vi "grabber_v2.vi"() -> ()   [LabVIEW 2010]
uses:
  <vilib>/Platform/TimedLoop/XDataNode/XDataNode.xnode
  <vilib>/Platform/TimedLoop/XDataNode/wakeup.ctl
  <vilib>/Platform/TimedLoop/XDataNode/XDNodeRunTimeDep.lvlib
  <vilib>/Platform/TimedLoop/XDataNode/nitl_modes.ctl
  <vilib>/Platform/TimedLoop/XDataNode/timing_clust.ctl
  <vilib>/rvi/interface/nirviCloseFPGA/nirviCloseFPGA.xnode
  <vilib>/rvi/interface/nirviMethod/nirviMethod.xnode
  <vilib>/rvi/interface/nirviReadWriteControl/nirviReadWriteControl.xnode
  <vilib>/Utility/error.llb/Error Cluster From Error Code.vi
  <vilib>/rvi/errors/niLvFpgaWhatHappensToTopLevelVI.ctl
  <vilib>/rvi/interface/common/niFpgaNodeNameForErrorReporting.ctl
  <vilib>/rvi/errors/niLvFpgaAdjustHostInterfaceError.vi
  <vilib>/dex/Flush And Wait Empty Condition.ctl
  NiFpgaLv.dll
  C:/Program Files (x86)/National Instruments/LabVIEW 2010/Targets/NI/FPGA/StockFPGA_IntfPrivate/ScriptTemplates/StockFPGA_ReadBigControlPlusUnflatten.vi
  <vilib>/FPGAPlugInAG/Dynamic/niLvFpga_Read32_Dynamic.vi
  C:/Program Files (x86)/National Instruments/LabVIEW 2010/Targets/NI/FPGA/StockFPGA_IntfPrivate/ScriptTemplates/StockFPGA_InlinedAdjustErrorForReadWrite.vi
  <vilib>/FPGAPlugInAG/Dynamic/niLvFpga_Close_Dynamic.vi
  config_data_cluster.ctl
panel:
  out "data lost":bool
  out "scan sum":T1
  out "y galvo feedback":i16(graph)
  out "x galvo feedback":i16(graph)
  out "z value":i16
  out "y value":i16
  out "x value":i16
  out "center of mass":cluster{"x avg":i16, "y avg":i16, "z avg":i16}
  in  "turn on displays":bool
  in  "Mark fly-forward phase?":bool
  in  "adjust N sums":u32=100 max=10000 step=20
  in  "fake image fast loop?":bool
  in  "Transpose graph view?":bool
  in  "Display green and red PMT?":bool
  in  "pick last TAG slice":u32
  in  "pick first TAG slice":u32
  in  "choose TAG slice?":bool
  out "ch1:position X":dbl
  out "ch0:position X":dbl
  in  "Adjust TAG phase":bool
  out "TAG profile at position X":dbl[][](graph)
  out "channel1":dbl[][](graph)
  out "channel0":dbl[][](graph)
  in  "N sums":u32(slide)=10 scale=0.0..100.0
  out "loop time":u32
  out "x galvo":i16(graph)
  out "scan specification":T2={"x amplitude"=100, "x resolution (pixels)"=28, "x offset fly-forward (iterations)"=50, "x offset fly-back (iterations)"=100, "y resolution (nr. of lines)"=80, "y step size"=30, "iterations per pixel"=5, "number of frames"=-1, "y offset (pixels)"=0, "number of y-brake lines  (before y-fly-back)"=0, "number y-brake lines (after y-fly-back)"=40, "number of y-fly-back steps"=0, "lines per z step"=1, "number of z/intensity tuples"=228, "number of repetitions (volumes or planes)"=-1, "z step size derived"=32, "choose the beginning of z scan"=FALSE, "number of frames (settings)"=80, "FPGA trajectory?"=TRUE, "Pockels cell voltage (bits)"=0, "Vy min(bits)"=0, "Vz min(bits)"=0}
  out "channel data block 2":dbl[][](graph)
  in  "fake image?":bool
  in  "xy view?":bool
  in  "Pockels cell voltage":i16(slide) min=-750 max=750 step=5 scale=-750.0..750.0
  out "DAC voltages":T3
  out "no. of extra wait lines written to FPGA FIFO":i32
  out "no. of z/int tuples written to FPGA FIFO":i32
  out "number of update commands received":i32
  out "extra wait lines set":bool
  out "zIntensity tuples set":bool
  out "scan spec set":bool
  out "display loop finished":bool
  in  "stop acquisition at FIFO overflow?  GRABBER":bool
  out "acquire?":bool
  out "FIFO overflow":bool
  out "scan":bool
  out "stop FPGA":bool
  out "wait for trigger?":bool
  out "stop acquisition at FIFO overflow?":bool
  out "scanning? FPGA":bool
  out "counter cluster out":T4
  out "extra waitlines array entries":u32[](graph)
  out "extra waitlines received by FPGA":u32
  out "no. of extra waitlines received":i32
  out "no of correctly transferred z tuples":u32
  out "z-points transfer corrupt?":bool
  out "intensity values":u16[](graph)
  out "z values":u16[](graph)
  out "no. of z/int. tubles received":i32
  out "z/intensity tuples received by FPGA":u32
  in  "wait till update":u32=500
  out "configuration":T5
  out "read FIFO overflow duration [ms]":u32
  out "read pixels duration [ms]":u32
  out "stream pixels [ms]":u32
  in  "Close front-panel?":bool=TRUE
  out "initialised?":bool
  in  "stop":bool
  out "command lp err":errorcluster
  out "error out":errorcluster
  out "effective read-block size":u32
  in  "max read block size":u32=32000
  out "read loop ctr":i32
  out "pixels read from FPGA":u64
  out "elements in FPGA FIFO":u32
  out "last received command":string
  out "command loop finished":bool
  out "read loop finished":bool
  out "scanning?":bool
  out "FIFO overflow?":bool
  out "data read from FPGA FIFO":u32[](array[numeric])
  # "enter a number between -+750V"
  # "Sum a single frame N times before displaying:"
  # "ms"
  # "automatically sets N=100 sums, otherwise FPGA buffer overflow"
  # "When T: displays and saves ch0.bin= green and ch1.bin =red\nWhen F: displays and saves ch0.bin= greenFF  and ch1.bin= greenFB  (FF=fly-forward and FB=fly-back)"
  # "Use when you want to display and save green and red PMT with marked FF and FB phases\nWhen T: fly-forward=photon counts+2^15 (number 1 at U16's most significant value)\n               and fly-back=photon counts\nWhen F: saves true photon count in both FF and FB phases of the red and green channel"
  # "How to use:\nTo adjust TAG phase\n1. set \"xy gavlo view?\"=F\n2. adjust Tag phase? = T\n3. drag cursor to desired x position\n   -- indicator below\n4. check z profile on the graph\n5. when done set N=0"
  # "How to use:\n1. set \"xy gavlo view?\"=T\n    on the main HS window\n2. to display xy view, sum all z stacks\n          set xy view?=T\n3. to choose a range of z slices to sum\na) xy view?=T\nb)choose TAG slice?=T\nc)eg. pick first Tag slice=3, pick last TAG slice=5\n   -> sums 3+4+5\nd) to display just one slice \n     set \"first=last\""
  # "RealTime Grabber"
  # "Status"
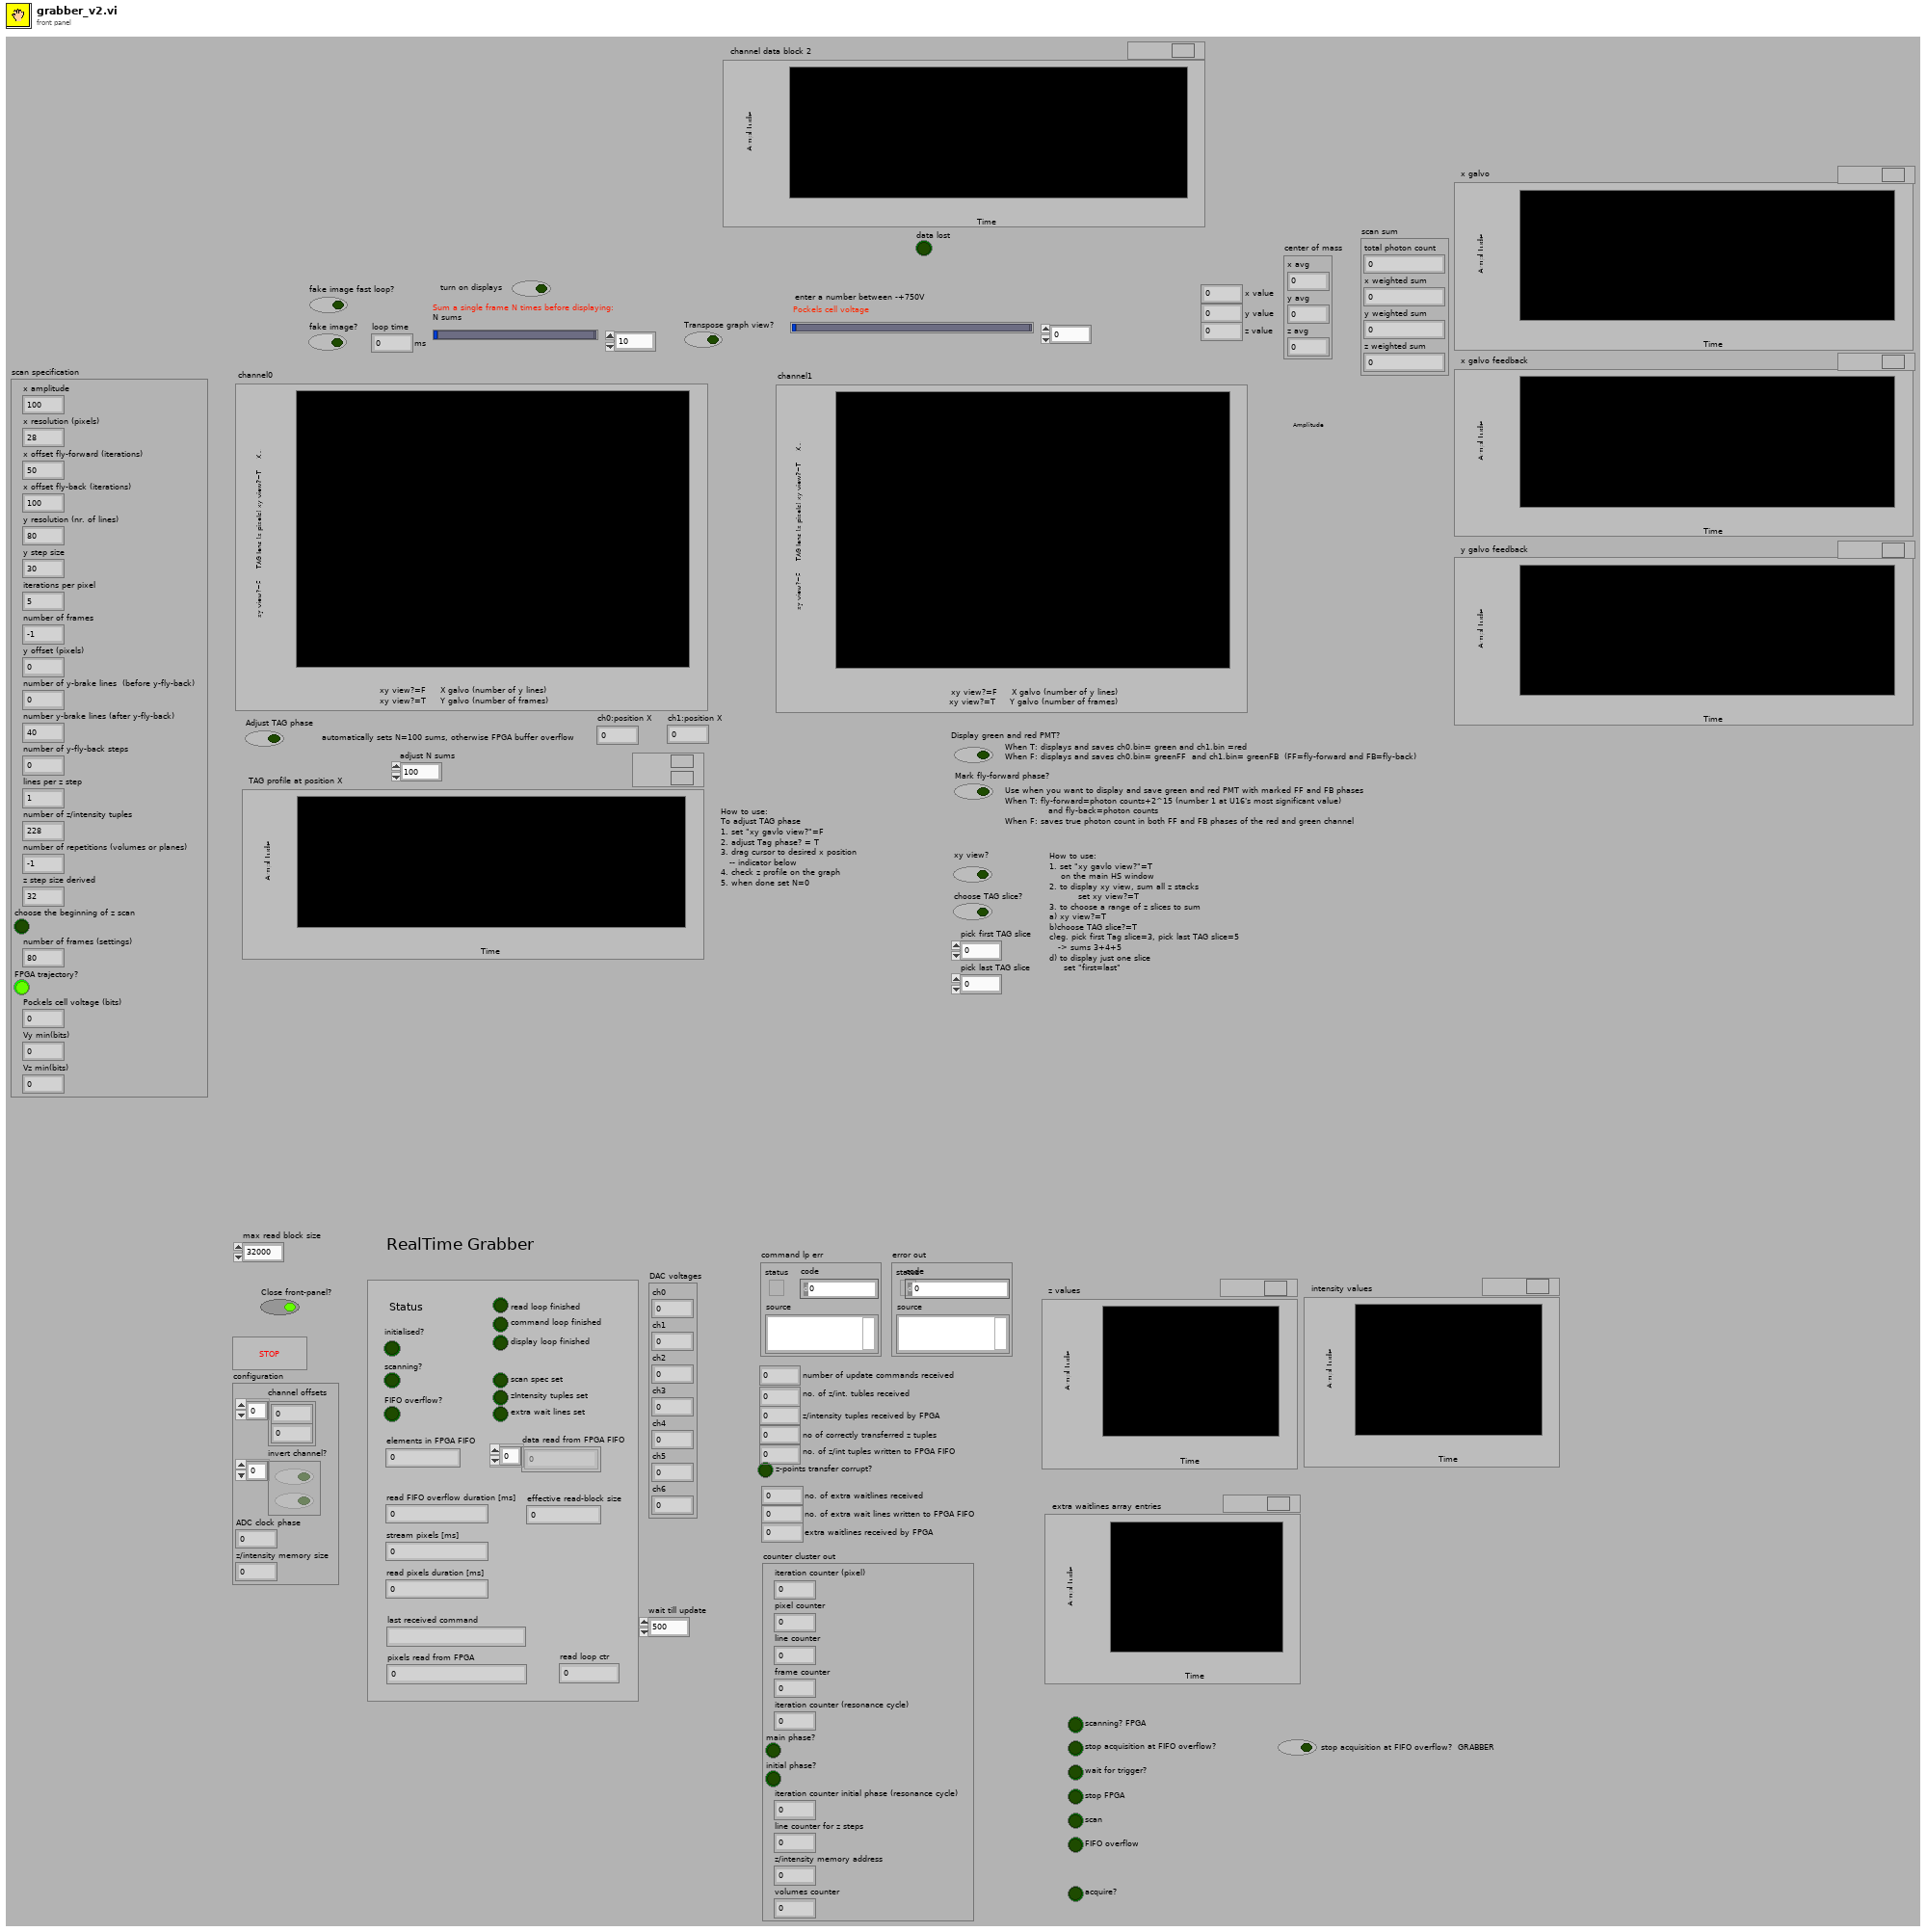
[diagram p1: front panel]
types:
  T1 = cluster{"total photon count":u64, "x weighted sum":i64, "y weighted sum":i64, "z weighted sum":i64}
  T2 = cluster{"x amplitude":u16, "x resolution (pixels)":u16, "x offset fly-forward (iterations)":u16, "x offset fly-back (iterations)":u16, "y resolution (nr. of lines)":u16, "y step size":u16, "iterations per pixel":u16, "number of frames":i32, "y offset (pixels)":u16, "number of y-brake lines  (before y-fly-back)":u16, "number y-brake lines (after y-fly-back)":u16, "number of y-fly-back steps":u16, "lines per z step":u16, "number of z/intensity tuples":u16, "number of repetitions (volumes or planes)":i32, "z step size derived":u16, "choose the beginning of z scan":bool, "number of frames (settings)":i32, "FPGA trajectory?":bool, "Pockels cell voltage (bits)":i16, "Vy min(bits)":i16, "Vz min(bits)":i16}
  T3 = cluster{"ch0":u16, "ch1":i16, "ch2":i16, "ch3":i16, "ch4":u16, "ch5":u16, "ch6":u16}
  T4 = cluster{"iteration counter (pixel)":u16, "pixel counter":u16, "line counter":u16, "frame counter":u16, "iteration counter (resonance cycle)":u16, "main phase?":bool, "initial phase?":bool, "iteration counter initial phase (resonance cycle)":u16, "line counter for z steps":u16, "z/intensity memory address":u32, "volumes counter":u16}
  T5 = typedef "config_data_cluster.ctl" = cluster{"channel offsets":u32[], "invert channel?":bool[], "ADC clock phase":i32, "z/intensity memory size":i32}
  T6 = cluster{"volumeQueue":refnum<queue>, "lineQueue":refnum<queue>, "comQueue":refnum<queue>}
  T7 = typedef "network_streaming_queues_cluster.ctl" = cluster{"data writer endpoint":refnum<k21>, "command reader endpoint":refnum<k21>, "settings reader endpoint":refnum<k21>, "z/intensity tuples reader endpoint":refnum<k21>, "extra waitlines reader endpoint":refnum<k21>}
  T8 = typedef "XDNodeRunTimeDep.lvlib/timing_clust.ctl" = cluster{"Expected End [f-1]":u64, "Actual End [f-1]":u64, "Finished Late? [f-1]":bool, "Expected End [i-1]":u64, "Actual End [i-1]":u64, "Finished Late? [i-1]":bool, "Expected Start [i]":u64, "Actual Start [i]":u64, "Expected Start [f]":u64, "Actual Start [f]":u64, "Source Name":string, "Structure Name":string, "Period":i64, "Deadline":i64, "Offset":i64, "Start":i64, "Priority":i32, "Timeout":i32, "Mode":T9, "Wakeup Reason":T10, "Error":errorcluster, "Source Type":string, "Secondary Source Type":string, "Global End Time":u64, "Global Start Time":u64, "Frame Duration":u64, "Iteration Duration":u64, "Assigned CPU":i32, "I/O Scan Engine Mode":u32}
  T9 = typedef "XDNodeRunTimeDep.lvlib/nitl_modes.ctl" = enum32{"No Change", "Process missed periods, maintain original phase", "Discard missed periods, maintain original phase", "Process missed periods, ignore original phase", "Discard missed periods, ignore original phase"}
  T10 = typedef "XDNodeRunTimeDep.lvlib/wakeup.ctl" = enum32{"Normal", "Aborted", "Asynchronous wakeup", "Timing source error", "Timed loop error", "Timeout"}
  T11 = typedef "niFpgaNodeNameForErrorReporting.ctl" = enum16{"Open FPGA VI Reference", "Read/Write Control", "Invoke Method: Abort", "Invoke Method: Acknowledge IRQ", "Invoke Method: Download", "Invoke Method: FIFO.Configure", "Invoke Method: FIFO.Read", "Invoke Method: FIFO.Start", "Invoke Method: FIFO.Stop", "Invoke Method: FIFO.Write", "Invoke Method: Reset", "Invoke Method: Run", "Invoke Method: Wait on IRQ", "Close FPGA VI Reference"}
  T12 = typedef "niLvFpgaWhatHappensToTopLevelVI.ctl" = enum16{"top level VI scripted behind XNode", "top level VI inlined behind XNode"}
  T13 = typedef "Flush And Wait Empty Condition.ctl" = u8
  T14 = typedef "scan_specification_cluster.ctl" = cluster{"x amplitude":u16, "x resolution (pixels)":u16, "x offset fly-forward (iterations)":u16, "x offset fly-back (iterations)":u16, "y resolution (nr. of lines)":u16, "y step size":u16, "iterations per pixel":u16, "number of frames":i32, "y offset (pixels)":u16, "number of y-brake lines  (before y-fly-back)":u16, "number y-brake lines (after y-fly-back)":u16, "number of y-fly-back steps":u16, "lines per z step":u16, "number of z/intensity tuples":u16, "number of repetitions (volumes or planes)":i32, "z step size derived":u16, "choose the beginning of z scan":bool, "number of frames (settings)":i32, "FPGA trajectory?":bool, "Pockels cell voltage (bits)":i16, "Vy min(bits)":i16, "Vz min(bits)":i16}
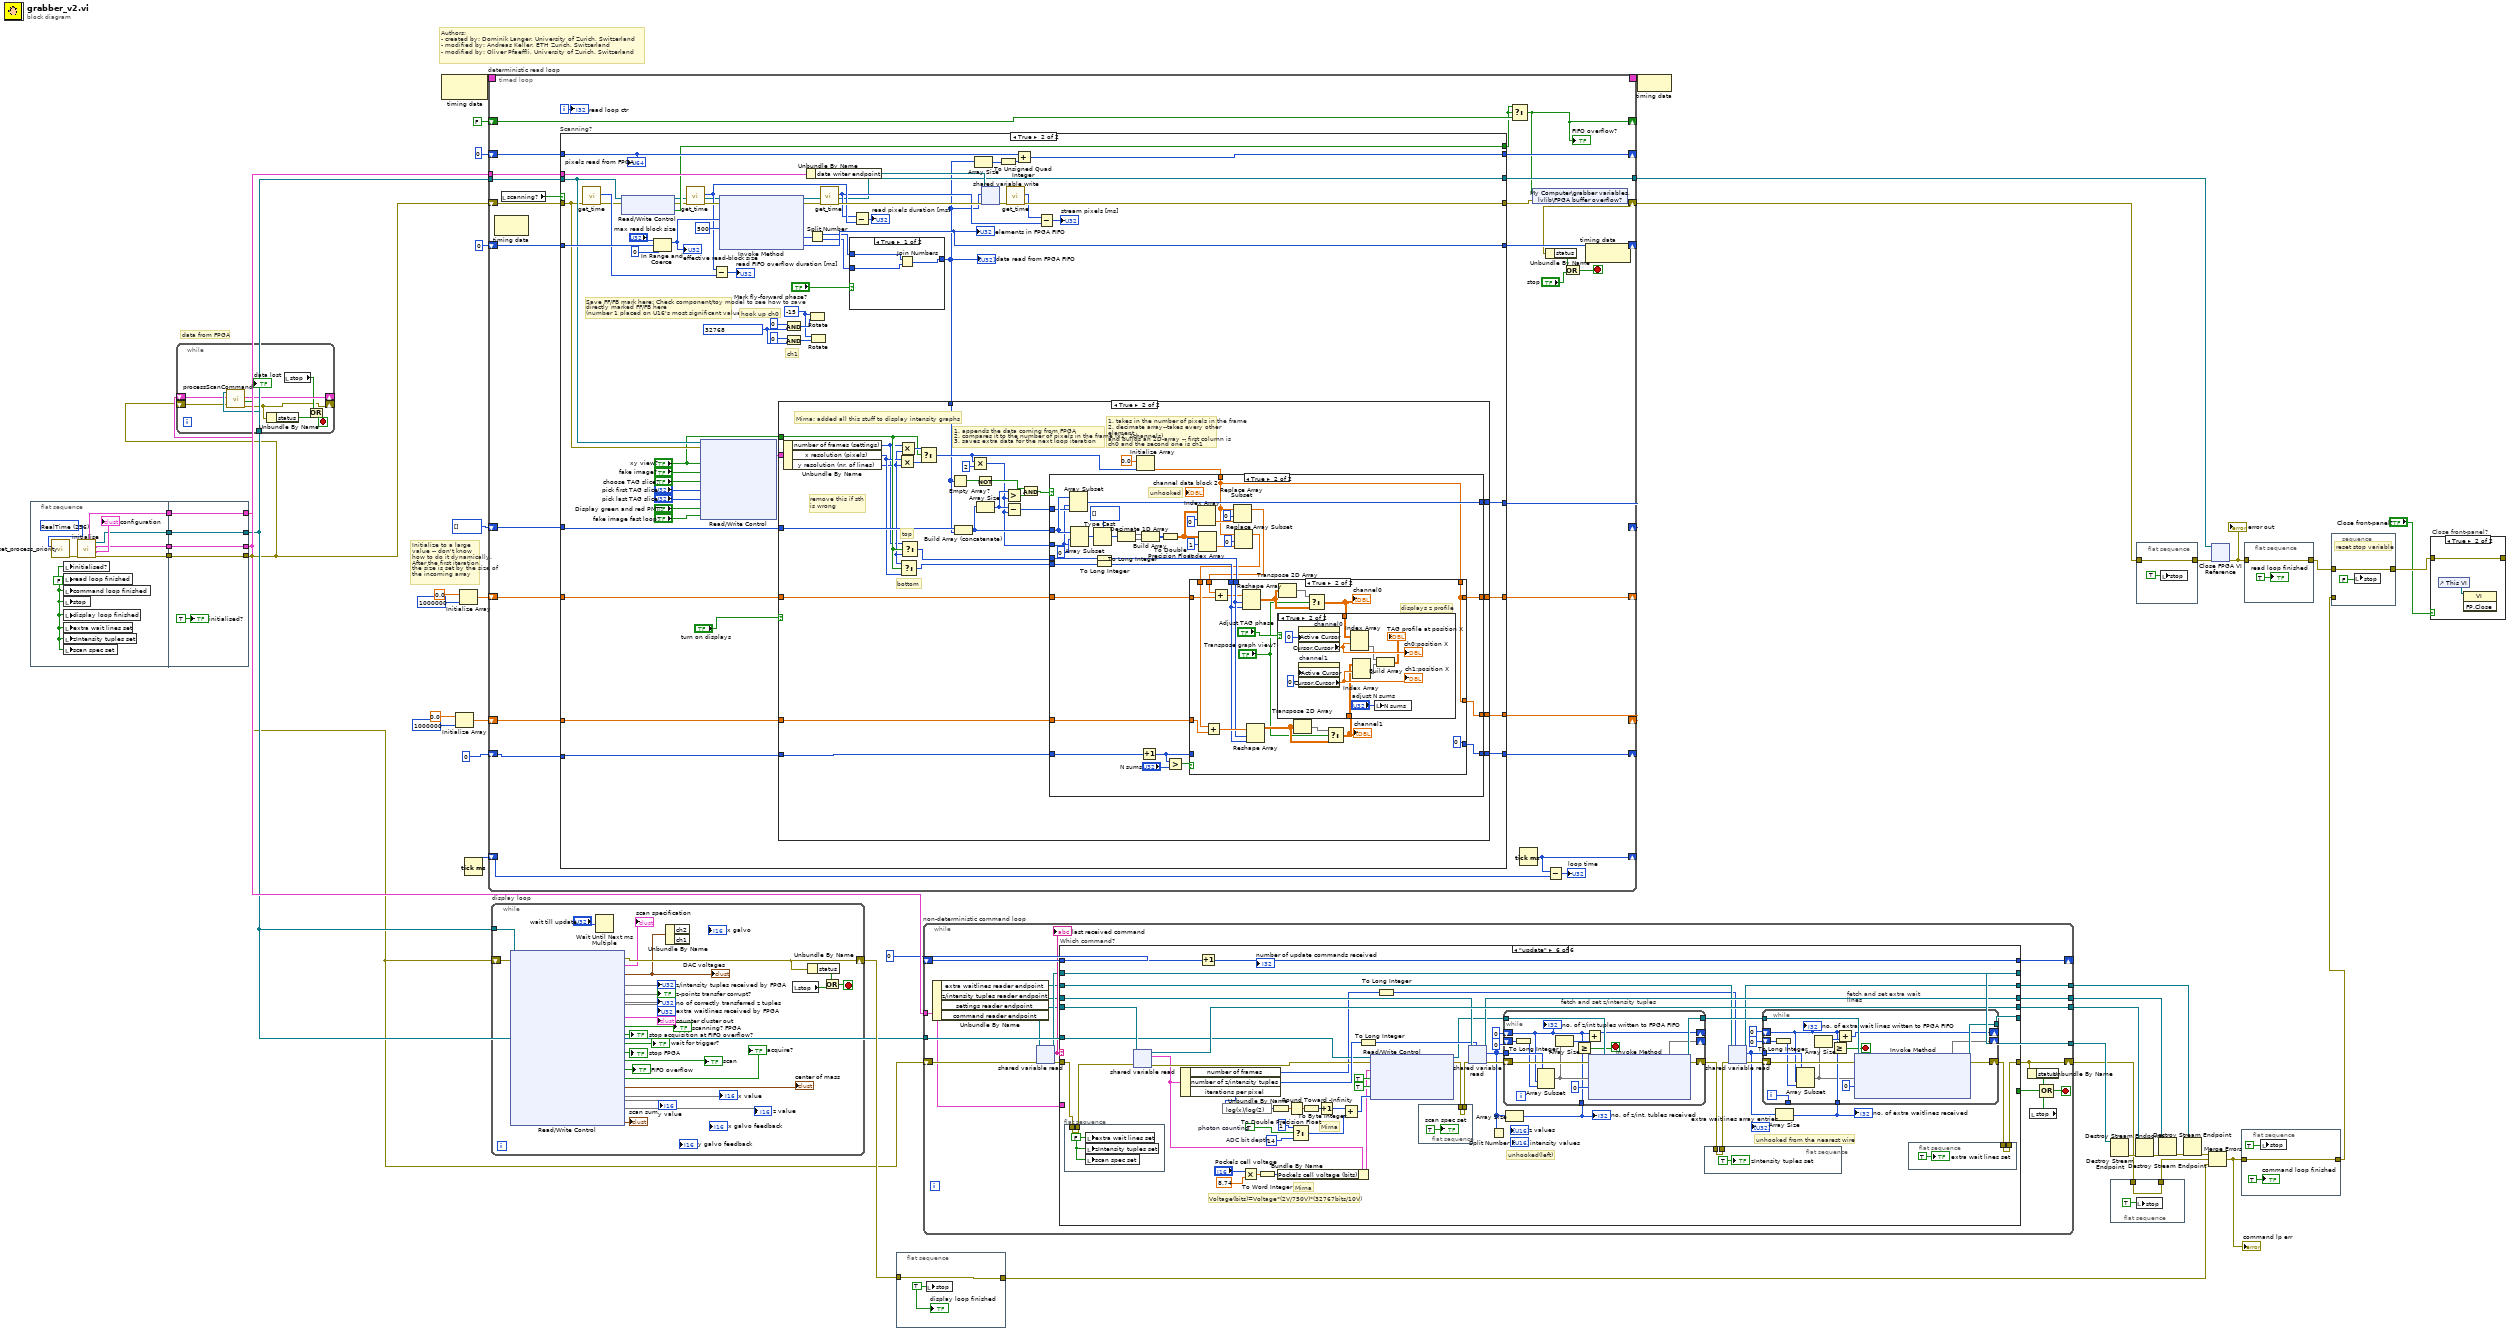
[diagram p0: block diagram]
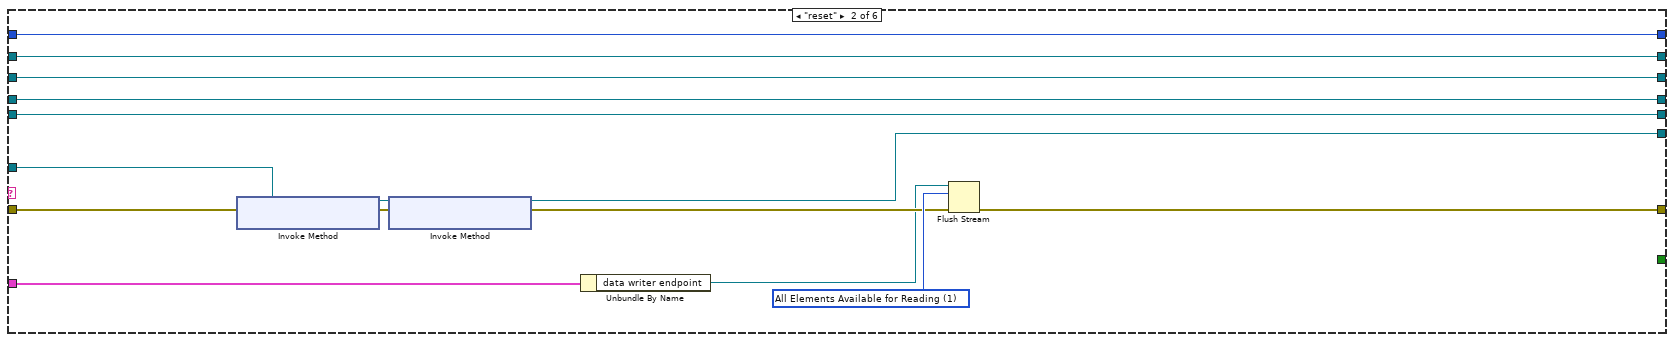
[diagram p4: hidden frame]
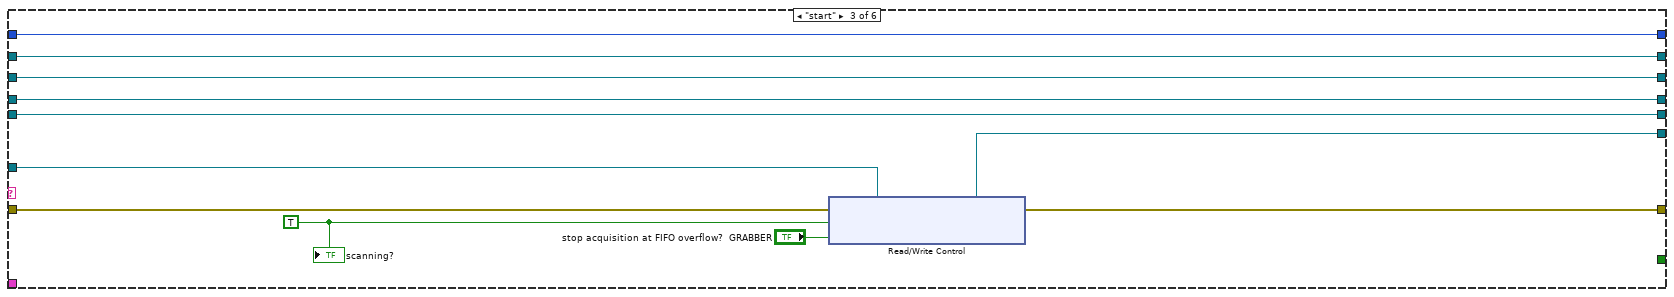
[diagram p5: hidden frame]
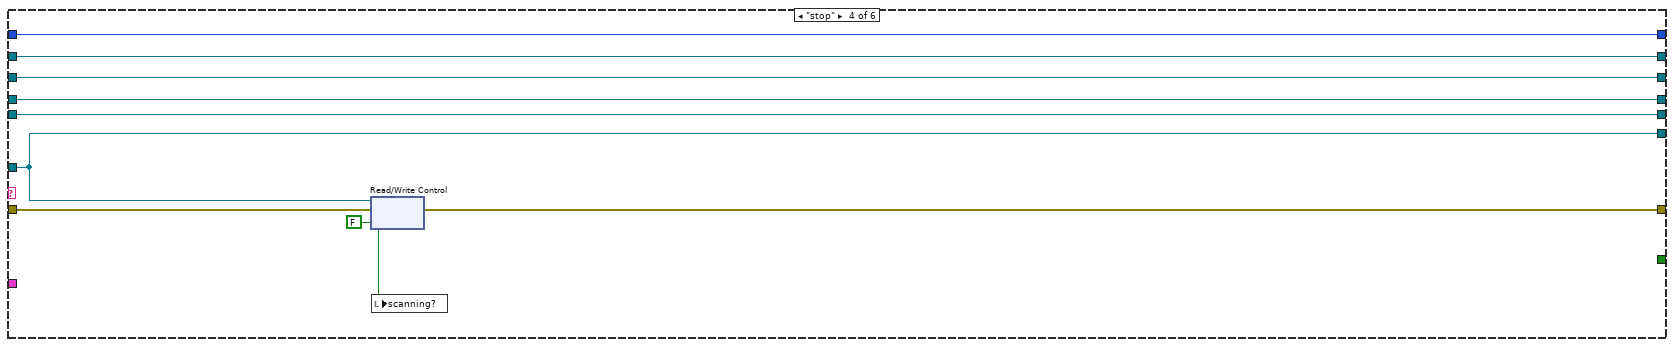
[diagram p6: hidden frame]
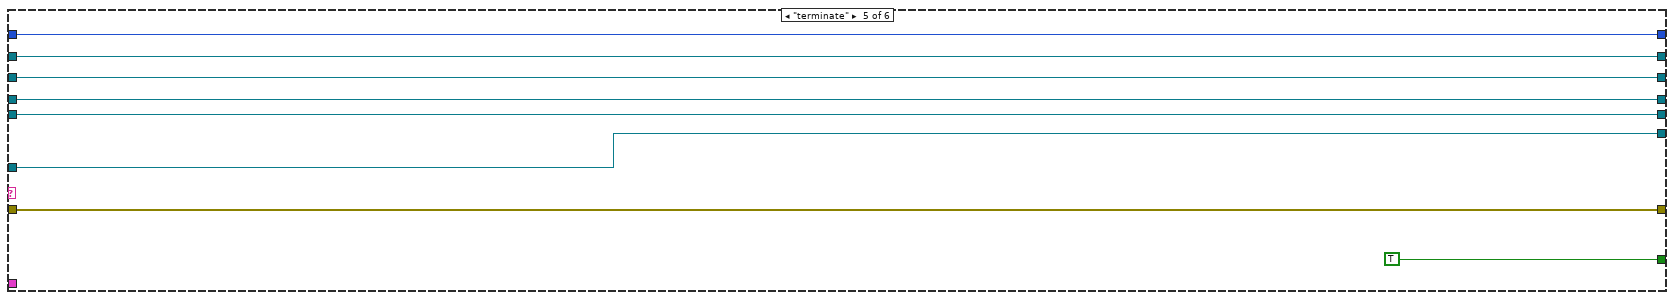
[diagram p7: hidden frame]
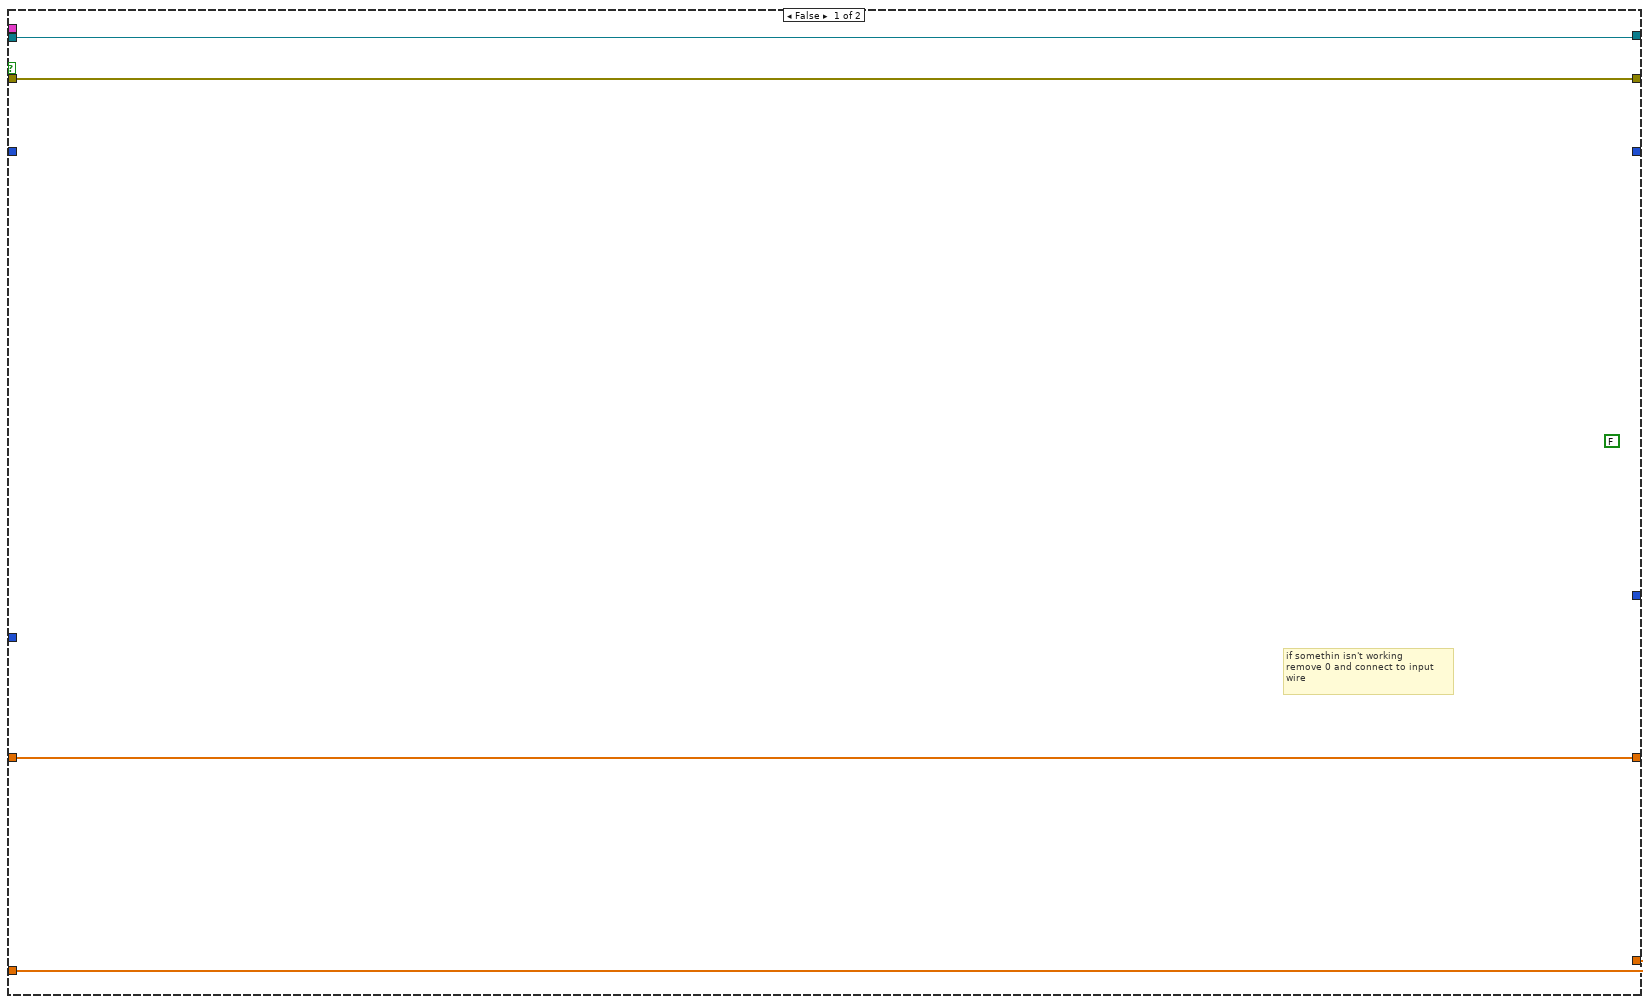
[diagram p8: hidden frame]
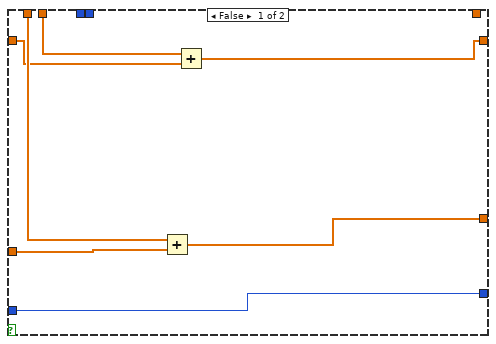
[diagram p11: hidden frame]
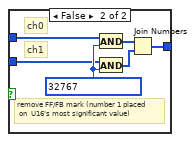
[diagram p13: hidden frame]
diagram:
  # "data from FPGA"
  # "Initialize to a large \nvalue -- don't know \nhow to do it dynamically.\nAfter the first iteration\nthe size is set by the size of\nthe incoming array"
  # "Authors: \n- created by: Dominik Langer, University of Zurich, Switzerland\n- modified by: Andreas Keller, ETH Zurich, Switzerland\n- modified by: Oliver Pfaeffli, University of Zurich, Switzerland"
  n1 = flat-sequence {
    tunnel: [w50] -> w35
    tunnel: [w47] -> w34
    tunnel: [w48] -> w31
    tunnel: [w45] -> w4
    tunnel: [w56] -> w2
    tunnel: [w57] -> w1
    tunnel: w35 -> [w57]
    tunnel: w34 -> [w56]
    tunnel: [w54] -> w30
    tunnel: w31 -> [w54]
    tunnel: [w53] -> w3
    tunnel: w4 -> [w53]
    frame #0 {
      w46 = FALSE ("read loop finished")
      w52 = 256 items=["Normal"=32, "Idle"=64, "High"=128, "RealTime"=256, "BelowNormal"=16384, "AboveNormal"=32768] ("PriorityClass")
      n2 = call "set_process_priority.vi"("PriorityClass"=w52) -> ("error out"=w51:errorcluster)  [unwired: 10 in]
      n3 = local write "initialised?"(w46) -> ()
      n4 = local write "read loop finished"(w46) -> ()
      n5 = local write "command loop finished"(w46) -> ()
      n6 = local write "stop"(w46) -> ()
      n7 = local write "display loop finished"(w46) -> ()
      n8 = local write "extra wait lines set"(w46) -> ()
      n9 = local write "zIntensity tuples set"(w46) -> ()
      n10 = local write "scan spec set"(w46) -> ()
      n11 = call "initialise.vi"("error in (no error)"=w51) -> ("Queues"=w45:T6, "error out"=w50:errorcluster, "configuration"=→"configuration":T5, "network streaming queues"=w48:T7, "FPGA VI Reference Out"=w47:refnum<k20>)  [unwired: 5 in]
    }
    frame #1 {
      "initialised?" <- TRUE ("initialised?")
    }
  }
  n12 = while {
    shift-right: [w66] -> _
    shift-left: w3 -> [w64]
    tunnel: w2 -> [w65]
    shift-right: [w58] -> _
    shift-left: w1 -> [w59]
    stop <- w60 stop-if-true
    n13 = call "processScanCommand.vi"("error in (no error)"=w59, "Queues"=w64, "FPGA VI Reference In"=w65) -> ("error out"=w58:errorcluster, "data lost"=→"data lost":bool, "Queues out"=w66:T6)  [unwired: 6 in]
    n14 = Unbundle By Name(w58) -> ("status"=w62:bool)
    n15 = local read "stop"() -> (w61:bool)
    n16 = Or(x=w61, y=w62) -> (x .or. y?=w60:bool)
  }
  n17 = node-c288 ("Input Node")() -> (w44:T8)  [unwired: 1 in]
  n18 = Initialize Array(0.0 ("element"), 1000000 ("dimension size")) -> (w12:dbl[])
  n19 = Initialize Array(0.0 ("element"), 1000000 ("dimension size")) -> (w6:dbl[])
  n20 = Tick Count (ms)() -> (millisecond timer value=w9:u32)
  n21 = timed-loop "deterministic read loop" {
    timing: w44 -> [_]
    timing-out: [_] -> w43
    shift-right: [w82] -> w24
    shift-left: w1 -> [w88]
    tunnel: w2 -> [w83]
    shift-right: [w69] -> _
    shift-left: FALSE ("FIFO overflow") -> [w95]
    shift-right: [w92] -> _
    shift-left: u64 0 -> [w94]
    tunnel: [w90] -> w37
    shift-right: [w86] -> _
    shift-left: u32 0 ("Elements Remaining") -> [w85]
    tunnel: w30 -> [w84]
    shift-right: [w77] -> _
    shift-left: u32[] [] -> [w78]
    shift-right: [w76] -> _
    shift-left: w12 -> [w75]
    shift-right: [w73] -> _
    shift-left: u32 0 ("Elements Remaining") -> [w74]
    shift-right: [w72] -> _
    shift-left: w9 -> [w71]
    shift-right: [w67] -> _
    shift-left: w6 -> [w68]
    i -> [w93]
    stop <- w79 stop-if-true
    n22 = node-c288 ("Output Node")() -> ()  [unwired: 1 in, 1 out]
    n23 = local read "scanning?"() -> (w87:bool)
    n24 = case "Scanning?" shown="True" w87 {
      tunnel: w88 -> [w101 w126]
      tunnel: [w101 w144] -> w89
      tunnel: w83 -> [w100 w130]
      tunnel: [w100 w132] -> w90
      tunnel: w94 -> [_ w152]
      tunnel: [_ w159] -> w92
      tunnel: [_ w135] -> w91
      tunnel: [_ w154] -> w86
      tunnel: w85 -> [_ w153]
      tunnel: w84 -> [_ w150]
      tunnel: w78 -> [_ w128]
      tunnel: [_ w127] -> w77
      tunnel: w75 -> [w98 w124]
      tunnel: [w98 w125] -> w76
      tunnel: w74 -> [_ w122]
      tunnel: [_ w123] -> w73
      tunnel: w68 -> [w99 w121]
      tunnel: [w99 w120] -> w67
      frame False {
        (unwired) FALSE ("FIFO overflow")
        # "if somethin isn't working \nremove 0 and connect to input \nwire"
      }
      frame True {
        w107 = i8 -15 ("y")
        w111 = u16 32768
        # "Save FF/FB mark here: Check component/toy model to see how to save directly marked FF/FB here\n(number 1 placed on U16's most significant value) FF=1, FB=0"
        # "ch1"
        # "hook up ch0"
        n25 = call "get_time.vi"("error in (no error)"=w126) -> ("error out"=w136:errorcluster, "millisecond timer value"=w140:u32)  [unwired: 9 in]
        n26 = xnode "Read/Write Control"("FPGA VI Reference In"=w130, "error in"=w136) -> ("FPGA VI Reference Out"=w133:refnum<k20>, "error out"=w134:errorcluster, "FIFO overflow"=w135:bool)
        n27 = In Range and Coerce(upper limit="max read block size", x=w153, lower limit=u32 0) -> (coerced(x)=w151:u32)  [unwired: 1 out]
        "effective read-block size" <- w151
        n28 = call "get_time.vi"("error in (no error)"=w134) -> ("error out"=w142:errorcluster, "millisecond timer value"=w138:u32)  [unwired: 9 in]
        n29 = xnode "Read/Write Control"("FPGA VI Reference In"=w130, "error in"=w126, "xy view?"="xy view?", "fake image?"="fake image?", "choose TAG slice?"="choose TAG slice?", "pick first TAG slice"="pick first TAG slice", "pick last TAG slice"="pick last TAG slice", "ch0-ch1?"="Display green and red PMT?", "fake image fast loop?"="fake image fast loop?") -> ("scan specification"=w131:T2)  [unwired: 2 out]
        n30 = Subtract(x=w138, y=w140) -> (x-y=→"read FIFO overflow duration [ms]":u32)
        n31 = xnode "Invoke Method"("FPGA VI Reference In"=w133, "error in"=w142, "Number of Elements"=w151, "Timeout (ms)"=500) -> ("FPGA VI Reference Out"=w132:refnum<k20>, "error out"=w147:errorcluster, "Data"=w114:u32[], "Elements Remaining"=w154:u32)
        "elements in FPGA FIFO" <- w154
        n32 = And(x=u16 0, y=w111) -> (x .and. y?=w109:u16)
        n33 = And(x=u16 0, y=w111) -> (x .and. y?=w108:u16)
        n34 = Unbundle By Name(w150) -> ("data writer endpoint"=w149:refnum<k21>)
        n35 = Split Number(x=w114) -> (hi(x)=w112:u16[], lo(x)=w110:u16[])
        n36 = Rotate(1:w109, 2:w107) -> ()  [unwired: 1 out]
        n37 = Rotate(1:w108, 2:w107) -> ()  [unwired: 1 out]
        n38 = call "get_time.vi"("error in (no error)"=w147) -> ("error out"=w146:errorcluster, "millisecond timer value"=w137:u32)  [unwired: 9 in]
        n39 = case shown="True" "Mark fly-forward phase?" {
          tunnel: [w268 w274] -> w113
          tunnel: w112 -> [w270 w272]
          tunnel: w110 -> [w269 w271]
          frame True {
            n40 = Join Numbers(hi=w270, lo=w269) -> ((hi.lo)=w268:u32[])
          }
          frame False {
            w276 = u16 32767
            # "ch1"
            # "ch0"
            # "remove FF/FB mark (number 1 placed\n on  U16's most significant value)"
            n41 = And(x=w272, y=w276) -> (x .and. y?=w275:u16[])
            n42 = And(x=w271, y=w276) -> (x .and. y?=w273:u16[])
            n43 = Join Numbers(hi=w275, lo=w273) -> ((hi.lo)=w274:u32[])
          }
        }
        "data read from FPGA FIFO" <- w113
        n44 = case shown="True" "turn on displays" {
          tunnel: w131 -> [_ w194]
          tunnel: w128 -> [w164 w184]
          tunnel: [w164 w183] -> w127
          tunnel: [w162 w178] -> w125
          tunnel: w124 -> [w162 w177]
          tunnel: [w161 w176] -> w123
          tunnel: w122 -> [w161 w175]
          tunnel: w121 -> [w163 w174]
          tunnel: [w163 w173] -> w120
          tunnel: "xy view?" -> [_ w172]
          tunnel: w113 -> [_ w167]
          frame False {
          }
          frame True {
            # "top"
            # "bottom"
            # "remove this if sth \nis wrong"
            # "1. takes in the number of pixels in the frame\n2. decimate array--takes every other element\nand builds an 2D-array -- first column is \nch0 and the second one is ch1"
            # "1. appends the data coming from FPGA\n2. compares it to the number of pixels in the frame (x2, 2channels)\n3. saves extra data for the next loop iteration"
            # "Mirna: added all this stuff to display intensity graphs"
            n45 = Unbundle By Name(w194) -> ("number of frames (settings)"=w166:i32, "x resolution (pixels)"=w170:u16, "y resolution (nr. of lines)"=w168:u16)
            n46 = Multiply(x=w170, y=w168) -> (x*y=w188:u16)
            n47 = Multiply(x=w166, y=w168) -> (x*y=w180:i32)
            n48 = Select(t=w168, s=w172, f=w170) -> (s? t:f=w171:u16)
            n49 = Select(t=w166, s=w172, f=w168) -> (s? t:f=w169:i32)
            n50 = Select(t=w180, s=w172, f=w188) -> (s? t:f=w181:i32)
            n51 = Empty Array?(array=w167) -> (empty?=w193:bool)
            n52 = Build Array (concatenate)(w184, w167) -> (w189:u32[])
            n53 = Multiply(x=w181, y=u16 2) -> (x*y=w185:i32)
            n54 = Not(x=w193) -> (.not. x?=w190:bool)
            n55 = Array Size(array=w189) -> (size(s)=w192:i32)
            n56 = Greater?(x=w192, y=w185) -> (0:w191:bool)
            n57 = Subtract(x=w192, y=w185) -> (x-y=w186:i32)
            n58 = And(x=w190, y=w191) -> (x .and. y?=w165:bool)
            n59 = Initialize Array(0.0 ("element"), w181) -> (w179:dbl[])
            n60 = case shown="True" w165 {
              tunnel: w189 -> [w198 w231]
              tunnel: w185 -> [_ w229]
              tunnel: w186 -> [_ w230]
              tunnel: [w198 w228] -> w183
              tunnel: w169 -> [_ w222]
              tunnel: w171 -> [_ w221]
              tunnel: w179 -> [_ w208]
              tunnel: w177 -> [w197 w214]
              tunnel: [w197 w209] -> w178
              tunnel: [w196 w213] -> w176
              tunnel: w175 -> [w196 w212]
              tunnel: w174 -> [w195 w203]
              tunnel: [w195 w202] -> w173
              frame False {
              }
              frame True {
                # "unhooked"
                n61 = Array Subset(array=w231, index=w229, length=w230) -> (w228:u32[])
                n62 = Array Subset(array=w231, index=0, length=w229) -> (w216:u32[])
                n63 = Type Cast(type=u16[] [], x=w216) -> (*(type *) &x=w225:u16[])
                n64 = To Long Integer(number=w222) -> (32bit integer=w207:i32)
                n65 = To Long Integer(number=w221) -> (32bit integer=w206:i32)
                n66 = Decimate 1D Array(w225) -> (w227:u16[], w226:u16[])
                n67 = Increment(x=w212) -> (x+1=w200:u32)
                n68 = Build Array(w227, w226) -> (w224:u16[][])
                n69 = To Double Precision Float(number=w224) -> (double precision float=w220:dbl[][])
                n70 = Greater?(x=w200, y="N sums") -> (0:w199:bool)
                n71 = Index Array(array=w220, index (row)=0) -> (element=w218:dbl[])  [unwired: 1 in]
                n72 = Index Array(array=w220, index (row)=1 ("index (col)")) -> (element=w210:dbl[])  [unwired: 1 in]
                n73 = Replace Array Subset(array=w208, new element=w218, index=0) -> (w204:dbl[])
                n74 = Replace Array Subset(array=w208, new element=w210, index=0) -> (w205:dbl[])
                n75 = case shown="True" w199 {
                  tunnel: w214 -> [w236 w257]
                  tunnel: [w239 u32 0] -> w213
                  tunnel: w205 -> [w238 w256]
                  tunnel: [w237 w249] -> w209
                  tunnel: w200 -> [w239 _]
                  tunnel: w208 -> [_ w249]
                  tunnel: w207 -> [_ w253]
                  tunnel: w206 -> [_ w252]
                  tunnel: w204 -> [w233 w251]
                  tunnel: w203 -> [w235 w250]
                  tunnel: [w234 w249] -> w202
                  frame False {
                    n76 = Add(x=w238, y=w236) -> (x+y=w237:dbl[])
                    n77 = Add(x=w233, y=w235) -> (x+y=w234:dbl[])
                  }
                  frame True {
                    # "displays z profile"
                    n78 = Add(x=w256, y=w257) -> (x+y=w254:dbl[])
                    n79 = Add(x=w251, y=w250) -> (x+y=w247:dbl[])
                    n80 = Reshape Array(w247, w253, w252) -> (w245:dbl[][])
                    n81 = Reshape Array(w254, w253, w252) -> (w242:dbl[][])
                    n82 = Transpose 2D Array(2D array=w245) -> (transposed array=w240:dbl[][])
                    n83 = Transpose 2D Array(2D array=w242) -> (transposed array=w244:dbl[][])
                    n84 = Select(t=w240, s="Transpose graph view?", f=w245) -> (s? t:f=w246:dbl[][])
                    "channel0" <- w246
                    n85 = Select(t=w244, s="Transpose graph view?", f=w242) -> (s? t:f=w243:dbl[][])
                    "channel1" <- w243
                    n86 = case shown="True" "Adjust TAG phase" {
                      tunnel: w246 -> [_ w266]
                      tunnel: w243 -> [_ w260]
                      frame False {
                      }
                      frame True {
                        n87 = property on="channel0" class="IntGraph (strict)"("Active Cursor"=u32 0) -> ("Cursor.Cursor X"=w265:dbl)  [unwired: 2 in, 2 out]
                        "ch0:position X" <- w265
                        n88 = property on="channel1" class="IntGraph (strict)"("Active Cursor"=u32 0) -> ("Cursor.Cursor X"=w263:dbl)  [unwired: 2 in, 2 out]
                        "ch1:position X" <- w263
                        n89 = Index Array(array=w266, index (row)=w265) -> (element=w262:dbl[])  [unwired: 1 in]
                        n90 = Index Array(array=w260, index (row)=w263) -> (element=w261:dbl[])  [unwired: 1 in]
                        n91 = local write "N sums"("adjust N sums") -> ()
                        n92 = Build Array(w262, w261) -> (→"TAG profile at position X":dbl[][])
                      }
                    }
                  }
                }
              }
            }
          }
        }
        n93 = Subtract(x=w137, y=w138) -> (x-y=→"read pixels duration [ms]":u32)
        n94 = Array Size(array=w113) -> (size(s)=w160:i32)
        n95 = shared-variable-write(w149, w146, w113) -> (w145:errorcluster)  [unwired: 1 in, 2 out]
        n96 = To Unsigned Quad Integer(1:w160) -> (0:w158:u64)
        n97 = call "get_time.vi"("error in (no error)"=w145) -> ("error out"=w144:errorcluster, "millisecond timer value"=w143:u32)  [unwired: 9 in]
        n98 = Add(x=w152, y=w158) -> (x+y=w159:u64)
        n99 = Subtract(x=w143, y=w137) -> (x-y=→"stream pixels [ms]":u32)
        "pixels read from FPGA" <- w152
      }
    }
    n100 = Select(t=w91, s=w91, f=w95) -> (s? t:f=w69:bool)
    "FIFO overflow?" <- w69
    n101 = Tick Count (ms)() -> (millisecond timer value=w72:u32)
    n102 = shared-variable "My Computer\\grabber variables.lvlib\\FPGA buffer overflow?"(w69, error in=w89) -> (error out=w82:errorcluster)
    n103 = Unbundle By Name(w82) -> ("status"=w81:bool)
    n104 = Subtract(x=w72, y=w71) -> (x-y=→"loop time":u32)
    n105 = Compound Arithmetic op=OR(w81, "stop") -> (w79:bool)
    n106 = node-c288 ("Input Node")() -> ()  [unwired: 1 in, 1 out]
    "read loop ctr" <- w93
  }
  n107 = while "display loop" {
    tunnel: w2 -> [w620]
    shift-right: [w618] -> w22
    shift-left: w1 -> [w619]
    stop <- w615 stop-if-true
    n108 = xnode "Read/Write Control"("FPGA VI Reference In"=w620, "error in"=w619) -> ("error out"=w618:errorcluster, "scan specification"=→"scan specification":T2, "DAC voltages"=w601:T3, "transferred z/intensity tuples"=→"z/intensity tuples received by FPGA", "z-points transfer corrupt?"=→"z-points transfer corrupt?", "no of correct transferred z tuples"=→"no of correctly transferred z tuples", "transferred extra waitlines"=→"extra waitlines received by FPGA", "counter cluster out"=→"counter cluster out":T4, "scanning?"=→"scanning? FPGA":bool, "stop acquisition at FIFO overflow?"=→"stop acquisition at FIFO overflow?":bool, "wait for trigger?"=→"wait for trigger?":bool, "stop"=→"stop FPGA":bool, "scan"=→"scan":bool, "FIFO overflow"=→"FIFO overflow":bool, "acquire?"=→"acquire?":bool, "center of mass"=→"center of mass":cluster{"x avg":i16, "y avg":i16, "z avg":i16}, "x value"=→"x value", "y value"=→"y value", "z value"=→"z value", "scan sum"=→"scan sum":T1)  [unwired: 1 out]
    "DAC voltages" <- w601
    n109 = Wait Until Next ms Multiple(millisecond multiple="wait till update") -> ()  [unwired: 1 out]
    n110 = Unbundle By Name(w601) -> ()  [unwired: 2 out]
    n111 = local read "stop"() -> (w616:bool)
    n112 = Unbundle By Name(w618) -> ("status"=w617:bool)
    n113 = Or(x=w617, y=w616) -> (x .or. y?=w615:bool)
  }
  n114 = flat-sequence {
    tunnel: w22 -> [w762]
    tunnel: [w762] -> w21
    frame #0 {
      w761 = TRUE ("stop")
      n115 = local write "stop"(w761) -> ()
      "display loop finished" <- w761
    }
  }
  n116 = while "non-deterministic command loop" {
    shift-right: [w770] -> w20
    shift-left: w1 -> [w783]
    tunnel: w2 -> [w782]
    tunnel: [w778] -> w42
    tunnel: w30 -> [w776]
    tunnel: [w774] -> w27
    tunnel: [w772] -> w25
    tunnel: [w765] -> w16
    shift-right: [w763] -> _
    shift-left: 0 -> [w764]
    stop <- w768 stop-if-true
    n117 = Unbundle By Name(w776) -> ("extra waitlines reader endpoint"=w766:refnum<k21>, "z/intensity tuples reader endpoint"=w773:refnum<k21>, "settings reader endpoint"=w775:refnum<k21>, "command reader endpoint"=w777:refnum<k21>)
    n118 = shared-variable-read(w777, w783) -> (w779:refnum<k21>, w781:errorcluster, w780:string)  [unwired: 1 in, 1 out]
    "last received command" <- w780
    n119 = case "Which command?" shown="\"update\"" w780 {
      tunnel: w782 -> [w788 w803 w858 w929 w976 w1017]
      tunnel: w781 -> [w790 w805 w856 w928 w975 w994]
      tunnel: [w790 w797 w860 w926 w975 w999] -> w770
      tunnel: w779 -> [w789 w804 w859 w930 w977 w1027]
      tunnel: [w789 w804 w859 w930 w977 w1027] -> w778
      tunnel: [w788 w802 w857 w929 w976 w1008] -> _
      tunnel: w776 -> [_ w796 _ _ _ _]
      tunnel: w775 -> [w787 w794 w854 w925 w974 w1026]
      tunnel: [w787 w794 w854 w925 w974 w1025] -> w774
      tunnel: w773 -> [w786 w793 w853 w924 w973 w1024]
      tunnel: [w786 w793 w853 w924 w973 w1023] -> w772
      tunnel: [_ _ _ _ TRUE _] -> w771
      tunnel: w766 -> [w785 w792 w852 w923 w971 w1006]
      tunnel: [w785 w792 w852 w923 w971 w1005] -> w765
      tunnel: w764 -> [w784 w791 w850 w922 w970 w992]
      tunnel: [w784 w791 w850 w922 w970 w991] -> w763
      frame "NULL", Default {
      }
      frame "reset" {
        w799 = T13 1 items=["All Elements Read From Stream", "All Elements Available for Reading"] ("wait condition")
        n120 = xnode "Invoke Method"("FPGA VI Reference In"=w803, "error in"=w805) -> ("FPGA VI Reference Out"=w800:refnum<k20>, "error out"=w801:errorcluster)
        n121 = xnode "Invoke Method"("FPGA VI Reference In"=w800, "error in"=w801) -> ("FPGA VI Reference Out"=w802:refnum<k20>, "error out"=w798:errorcluster)
        n122 = Unbundle By Name(w796) -> ("data writer endpoint"=w795:refnum<k21>)
        n123 = Flush Stream(8:w798, 10:w799, 11:w795) -> (0:w797:errorcluster)  [unwired: 1 in, 2 out]
      }
      frame "start" {
        w855 = TRUE ("scan")
        n124 = xnode "Read/Write Control"("FPGA VI Reference In"=w858, "error in"=w856, "scan"=w855, "stop acquisition at FIFO overflow?"="stop acquisition at FIFO overflow?  GRABBER") -> ("FPGA VI Reference Out"=w857:refnum<k20>, "error out"=w860:errorcluster)
        "scanning?" <- w855
      }
      frame "stop" {
        w927 = FALSE ("scan")
        n125 = xnode "Read/Write Control"("FPGA VI Reference In"=w929, "error in"=w928, "scan"=w927) -> ("error out"=w926:errorcluster)  [unwired: 1 out]
        n126 = local write "scanning?"(w927) -> ()
      }
      frame "terminate" {
      }
      frame "update" {
        w986 = TRUE  # photon counting
        w990 = i8 14  # ADC bit depth
        # "unhooked from the nearest wire"
        # "unhooked(left)"
        # "Mirna"
        # "Voltage(bits)=Voltage*(2V/750V)*(32767bits/10V)"
        # "Mirna"
        n127 = flat-sequence {
          tunnel: w994 -> [w1033]
          tunnel: [w1033] -> w993
          frame #0 {
            w1034 = FALSE ("extra wait lines set")
            n128 = local write "extra wait lines set"(w1034) -> ()
            n129 = local write "zIntensity tuples set"(w1034) -> ()
            n130 = local write "scan spec set"(w1034) -> ()
          }
        }
        n131 = shared-variable-read(w1026, w993) -> (w1025:refnum<k21>, w1019:errorcluster, w981:T14)  [unwired: 1 in, 1 out]
        n132 = Unbundle By Name(w981) -> ("number of frames"=w1004:i32, "number of z/intensity tuples"=w1022:u16, "iterations per pixel"=w980:u16)
        n133 = Increment(x=w992) -> (x+1=w991:i32)
        "number of update commands received" <- w991
        n134 = expression code="log(x)/log(2)"(w980) -> (w1028:u16)
        n135 = Multiply(x="Pockels cell voltage", y=8.74 ("x")) -> (x*y=w983:dbl)
        n136 = To Word Integer(number=w983) -> (16bit integer=w982:i16)
        n137 = To Double Precision Float(number=w1028) -> (double precision float=w1030:dbl)
        n138 = Bundle By Name(cluster=w981, "Pockels cell voltage (bits)"=w982) -> (w979:T14)
        n139 = Round Toward -Infinity(1:w1030) -> (0:w1029:dbl)
        n140 = Select(t=i8 1, s=w986, f=w990) -> (s? t:f=w988:i8)
        n141 = To Byte Integer(number=w1029) -> (8bit integer=w1031:i8)
        n142 = Increment(x=w1031) -> (x+1=w1032:i8)
        n143 = Add(x=w1032, y=w988) -> (x+y=w1012:i8)
        n144 = To Long Integer(number=w1022) -> (32bit integer=w1021:i32)
        n145 = xnode "Read/Write Control"("FPGA VI Reference In"=w1017, "error in"=w1019, "scan specification"=w979, "transfer z-points?"=TRUE, "transfer extra-waitlines?"=TRUE ("transfer z-points?"), "maximum bit depth"=w1012) -> ("FPGA VI Reference Out"=w1018:refnum<k20>, "error out"=w996:errorcluster)
        n146 = To Long Integer(number=w1004) -> (32bit integer=w1003:i32)
        n147 = flat-sequence {
          tunnel: [w1039] -> w995
          tunnel: w996 -> [w1039]
          frame #0 {
            "scan spec set" <- TRUE ("zIntensity tuples set")
          }
        }
        n148 = shared-variable-read(w1024, w995, w1021) -> (w1023:refnum<k21>, w1020:errorcluster, w1016:u32[])  [unwired: 1 in, 1 out]
        n149 = Split Number(x=w1016) -> ()  [unwired: 2 out]
        n150 = Array Size(array=w1016) -> (size(s)=w1015:i32)
        "no. of z/int. tubles received" <- w1015
        n151 = while "fetch and set z/intensity tuples" {
          tunnel: [w1072] -> w1009
          tunnel: w1018 -> [w1071]
          shift-right: [w1069] -> _
          shift-left: u32 0 ("Empty Elements Remaining") -> [w1067]
          tunnel: w1016 -> [w1068]
          shift-right: [w1065] -> _
          shift-left: 0 -> [w1062]
          tunnel: w1015 -> [w1061]
          shift-right: [w1073] -> w998
          shift-left: w1020 -> [w1074]
          stop <- w1060 stop-if-true
          n152 = To Long Integer(number=w1067) -> (32bit integer=w1066:i32)
          n153 = Array Subset(array=w1068, index=w1062, length=w1066) -> (w1063:u32[])
          n154 = Array Size(array=w1063) -> (size(s)=w1064:i32)
          n155 = Greater Or Equal?(x=w1062, y=w1061) -> (x >= y?=w1060:bool)
          n156 = Add(x=w1062, y=w1064) -> (x+y=w1065:i32)
          n157 = xnode "Invoke Method"("FPGA VI Reference In"=w1071, "error in"=w1074, "Data"=w1063, "Timeout (ms)"=0) -> ("FPGA VI Reference Out"=w1072:refnum<k20>, "error out"=w1073:errorcluster, "Empty Elements Remaining"=w1069)
          "no. of z/int tuples written to FPGA FIFO" <- w1062
        }
        n158 = flat-sequence {
          tunnel: [w1037] -> w997
          tunnel: w998 -> [w1037]
          frame #0 {
            "zIntensity tuples set" <- TRUE ("scan spec set")
          }
        }
        n159 = shared-variable-read(w1006, w997, w1003) -> (w1005:refnum<k21>, w1007:errorcluster, w978:u32[])  [unwired: 1 in, 1 out]
        n160 = Array Size(array=w978) -> (size(s)=w1002:i32)
        "no. of extra waitlines received" <- w1002
        n161 = while "fetch and set extra wait lines" {
          shift-right: [w1045] -> _
          shift-left: 0 -> [w1042]
          shift-right: [w1046] -> _
          shift-left: u32 0 ("Empty Elements Remaining") -> [w1051]
          tunnel: w1009 -> [w1056]
          tunnel: [w1055] -> w1008
          tunnel: w978 -> [w1052]
          tunnel: w1002 -> [w1048]
          shift-right: [w1053] -> w1000
          shift-left: w1007 -> [w1054]
          tunnel: [w1041] -> _
          i -> [w1041]
          stop <- w1047 stop-if-true
          n162 = To Long Integer(number=w1051) -> (32bit integer=w1050:i32)
          n163 = Array Subset(array=w1052, index=w1042, length=w1050) -> (w1044:u32[])
          n164 = Array Size(array=w1044) -> (size(s)=w1049:i32)
          n165 = Greater Or Equal?(x=w1042, y=w1048) -> (x >= y?=w1047:bool)
          n166 = Add(x=w1042, y=w1049) -> (x+y=w1045:i32)
          n167 = xnode "Invoke Method"("FPGA VI Reference In"=w1056, "error in"=w1054, "Data"=w1044, "Timeout (ms)"=0) -> ("FPGA VI Reference Out"=w1055:refnum<k20>, "error out"=w1053:errorcluster, "Empty Elements Remaining"=w1046)
          "no. of extra wait lines written to FPGA FIFO" <- w1042
        }
        n168 = flat-sequence {
          tunnel: w1000 -> [w1035]
          tunnel: [w1035] -> w999
          frame #0 {
            "extra wait lines set" <- TRUE ("extra wait lines set")
          }
        }
      }
    }
    n169 = Unbundle By Name(w770) -> ("status"=w769:bool)
    n170 = local read "stop"() -> (w767:bool)
    n171 = Compound Arithmetic op=OR(w769, w771, w767) -> (w768:bool)
  }
  n172 = node-c288 ("Output Node")(w43) -> ()
  n173 = Destroy Stream Endpoint(11:w42) -> (0:w28:errorcluster)  [unwired: 1 in]
  n174 = flat-sequence {
    tunnel: [w1197] -> w19
    tunnel: w20 -> [w1197]
    frame #0 {
      n175 = local write "stop"(TRUE ("stop")) -> ()
    }
  }
  n176 = Destroy Stream Endpoint(8:w28, 11:w27) -> (0:w26:errorcluster)
  n177 = flat-sequence {
    tunnel: w24 -> [w1199]
    tunnel: [w1199] -> w23
    frame #0 {
      n178 = local write "stop"(TRUE ("stop")) -> ()
    }
  }
  n179 = Destroy Stream Endpoint(8:w26, 11:w25) -> (0:w18:errorcluster)
  n180 = Destroy Stream Endpoint(8:w18, 11:w16) -> (0:w17:errorcluster)
  n181 = Merge Errors(w17, w19, w21) -> (w36:errorcluster)
  "command lp err" <- w36
  n182 = xnode "Close FPGA VI Reference"("FPGA VI Reference In"=w37, "error in"=w23) -> ("error out"=w29:errorcluster)
  "error out" <- w29
  n183 = flat-sequence {
    tunnel: w36 -> [w1201]
    tunnel: [w1201] -> w41
    frame #0 {
      n184 = local write "stop"(TRUE ("stop - RT")) -> ()
      "command loop finished" <- TRUE ("command loop finished")
    }
  }
  n185 = flat-sequence {
    tunnel: w29 -> [w1205]
    tunnel: [w1205] -> w40
    frame #0 {
      "read loop finished" <- TRUE ("read loop finished")
    }
  }
  n186 = stacked-sequence {
    tunnel: w41 -> [_]
    tunnel: w40 -> [w1206]
    tunnel: [w1206] -> w33
    frame #0 {
      # "reset stop variable"
      n187 = local write "stop"(FALSE) -> ()
    }
  }
  n188 = case "Close front-panel?" shown="True" "Close front-panel?" {
    tunnel: [w1208 w1209] -> _
    tunnel: w33 -> [w1208 w1209]
    frame False {
    }
    frame True {
      n189 = control-ref of="This VI"() -> (w1210:refnum<vi>)
      n190 = invoke class="VI" method="FP.Close"(reference=w1210) -> ()  [unwired: 2 in, 3 out]
    }
  }
